vi "test_led.vi"() -> ()   [LabVIEW 2019]
panel:
  out "output array":bool[](array[boolean])
  out "appended array":bool[](array[boolean])=[TRUE, FALSE, TRUE]
  in  "stop":bool
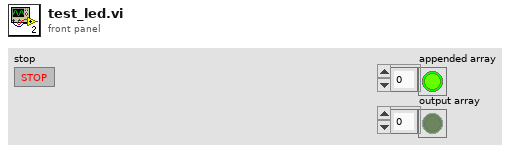
[diagram p1: front panel]
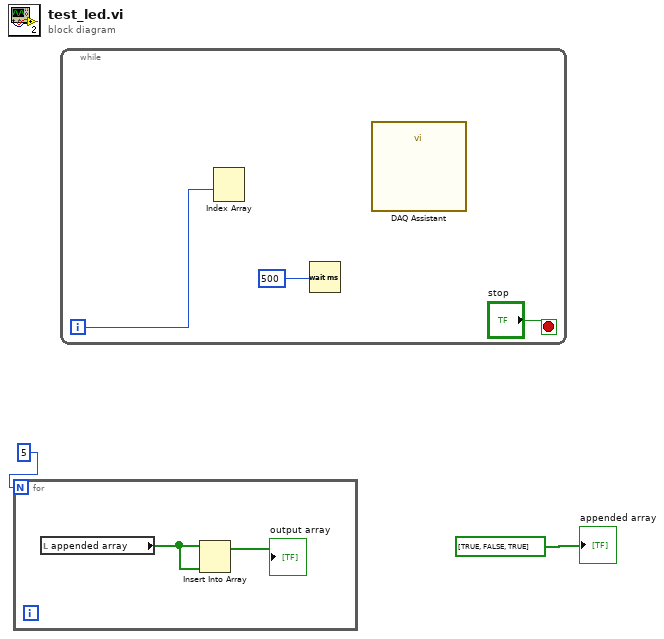
[diagram p0: block diagram]
diagram:
  n1 = for {
    N: 5 -> [_]
    n2 = local read "appended array"() -> (w4:bool[])
    n3 = Insert Into Array(array=w4, new element=w4) -> (→"output array":bool[])  [unwired: 1 in]
  }
  n4 = while {
    i -> [w7]
    stop <- "stop" stop-if-true
    n5 = Index Array(index (row)=w7) -> ()  [unwired: 2 in, 1 out]
    n6 = Wait (ms)(milliseconds to wait=500) -> ()  [unwired: 1 out]
    n7 = call "DAQ Assistant"() -> ()  [unwired: 18 in, 2 out]
  }
  "appended array" <- bool[] [TRUE, FALSE, TRUE] ("appended array")
